vi "cal_para.vi"() -> (3 "std sample":T1(array[cluster]))   [LabVIEW 2013]
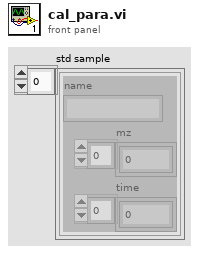
[diagram p1: front panel]
types:
  T1 = cluster{"name":string, "mz":dbl[], "time":dbl[]}[]
  T2 = cluster{"name":string, "mz":dbl[], "tof":dbl[]}[]
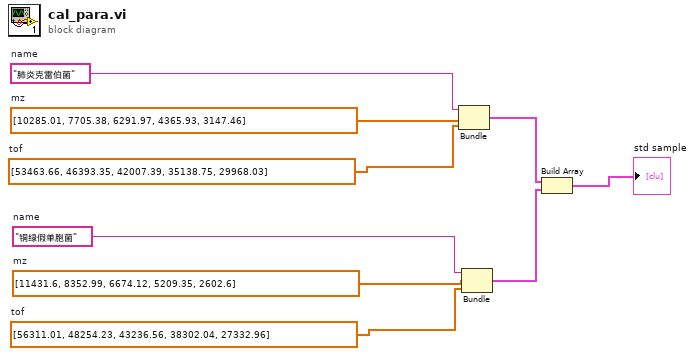
[diagram p0: block diagram]
diagram:
  w4 = dbl[] [56311.01, 48254.23, 43236.56, 38302.04, 27332.96]  # tof
  w5 = dbl[] [11431.6, 8352.99, 6674.12, 5209.35, 2602.6]  # mz
  w6 = "铜绿假单胞菌"  # name
  w7 = dbl[] [53463.66, 46393.35, 42007.39, 35138.75, 29968.03]  # tof
  w8 = dbl[] [10285.01, 7705.38, 6291.97, 4365.93, 3147.46]  # mz
  w9 = "肺炎克雷伯菌"  # name
  n1 = Bundle("name"=w9, "mz"=w8, "tof"=w7) -> (w3:cluster{"name":string, "mz":dbl[], "tof":dbl[]})  [unwired: 1 in]
  n2 = Bundle("name"=w6, "mz"=w5, "tof"=w4) -> (w2:cluster{"name":string, "mz":dbl[], "tof":dbl[]})  [unwired: 1 in]
  n3 = Build Array(w3, w2) -> (→"std sample":T2)
